vi "Save File DOE Seperate Scan List By Agilent.vi"(10 "TC Channel-List":string[](array[string]), 11 "Analog Channel-List":string[](array[string])) -> (0 "TC List Agilent 2":string, 1 "TC List Agilent 1":string, 2 "Analog Channel-List 2":string, 3 "Analog Channel-List 1":string)   [LabVIEW 2020, in "File Setup.lvlib"]
uses:
  File Setup.lvlib
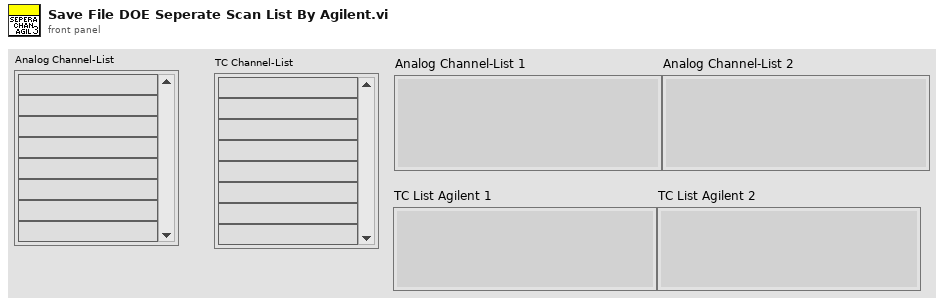
[diagram p1: front panel]
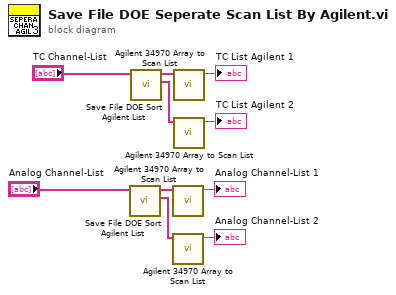
[diagram p0: block diagram]
diagram:
  n1 = call "Save File DOE Sort Agilent List.vi"("TC Channel-List"="Analog Channel-List") -> ("TC List Agilent 2"=w1:string[], "TC List Agilent 1"=w2:string[])  [unwired: 9 in]
  n2 = call "Save File DOE Sort Agilent List.vi"("TC Channel-List"="TC Channel-List") -> ("TC List Agilent 2"=w5:string[], "TC List Agilent 1"=w8:string[])  [unwired: 9 in]
  n3 = call "Agilent 34970 Array to Scan List.vi"("Agilent Channels (Temperature TC)"=w2) -> ("Agilent Scan List"=→"Analog Channel-List 1":string)  [unwired: 10 in]
  n4 = call "Agilent 34970 Array to Scan List.vi"("Agilent Channels (Temperature TC)"=w1) -> ("Agilent Scan List"=→"Analog Channel-List 2":string)  [unwired: 10 in]
  n5 = call "Agilent 34970 Array to Scan List.vi"("Agilent Channels (Temperature TC)"=w8) -> ("Agilent Scan List"=→"TC List Agilent 1":string)  [unwired: 10 in]
  n6 = call "Agilent 34970 Array to Scan List.vi"("Agilent Channels (Temperature TC)"=w5) -> ("Agilent Scan List"=→"TC List Agilent 2":string)  [unwired: 10 in]
